vi "Write azElParameters.vi"(8 "error in (no error)":errorcluster, 10 "AzElParameters.lvclass":refnum<class "AzElParameters.lvclass">, 11 "AzElTarget in":refnum<class "AzElTarget.lvclass">) -> (0 "error out":errorcluster, 3 "AzElTarget out":refnum<class "AzElTarget.lvclass">)   [LabVIEW 2022 SP3, in "TCSDataDefinitions.lvlib" / "TCSCommand.lvlib" / "TargetConfiguration.lvlib" / "Target.lvlib" / "FixedTarget.lvlib" / "AzElTarget.lvclass"]
uses:
  AzElTarget.lvclass
  AzElParameters/AzElParameters.lvclass
  AzElTarget.lvclass/AzElTarget.ctl
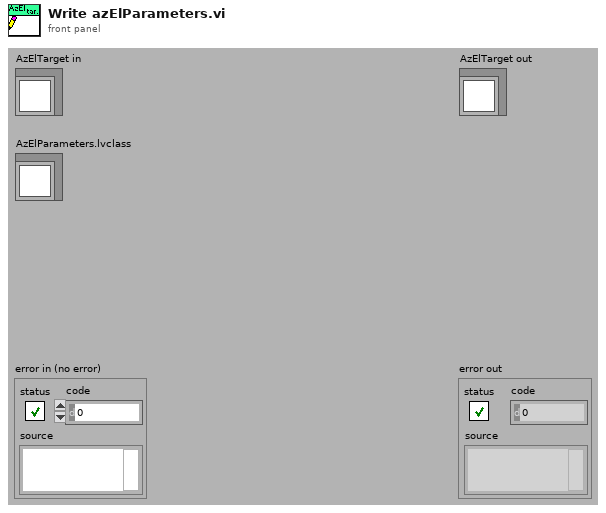
[diagram p1: front panel]
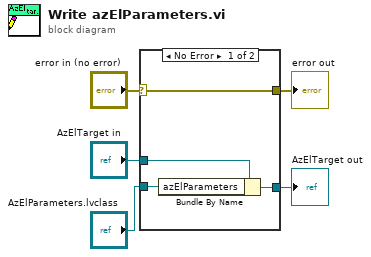
[diagram p0: block diagram]
diagram:
  n1 = case shown="No Error" "error in (no error)" {
    selector: "error in (no error)" -> [w9 w10]
    tunnel: [w9 w10] -> w4
    tunnel: [w7 w11] -> w2
    tunnel: "AzElTarget in" -> [w8 w11]
    tunnel: "AzElParameters.lvclass" -> [w6 _]
    frame No Error {
      n2 = Bundle By Name(cluster=w8, "azElParameters"=w6) -> (w7:refnum<class "AzElTarget.lvclass">)
    }
    frame Error {
    }
  }
  "error out" <- w4
  "AzElTarget out" <- w2
